vi "FMA1600A Meter Present.vi"(7 "Unit ID":string, 8 "error in (no error)":errorcluster, 9 "Meter Present":bool, 10 "Data Frame Format In":T2, 11 "VISA Refnum in":refnum<visa-resource-name>) -> (0 "error out":errorcluster, 2 "FMA1600A Gas Data":T3, 3 "Data Cluster":T1)   [LabVIEW 2023]
uses:
  Type Definitions/FMA1600A Data.ctl
  Alicat Gas Meter Driver/Sub-VIs/Data Frame.ctl
  Alicat Gas Meter Driver/Sub-VIs/Data Cluster.ctl
  Type Definitions/FMA1600A Commands.ctl
panel:
  # "Totalizer Timer"
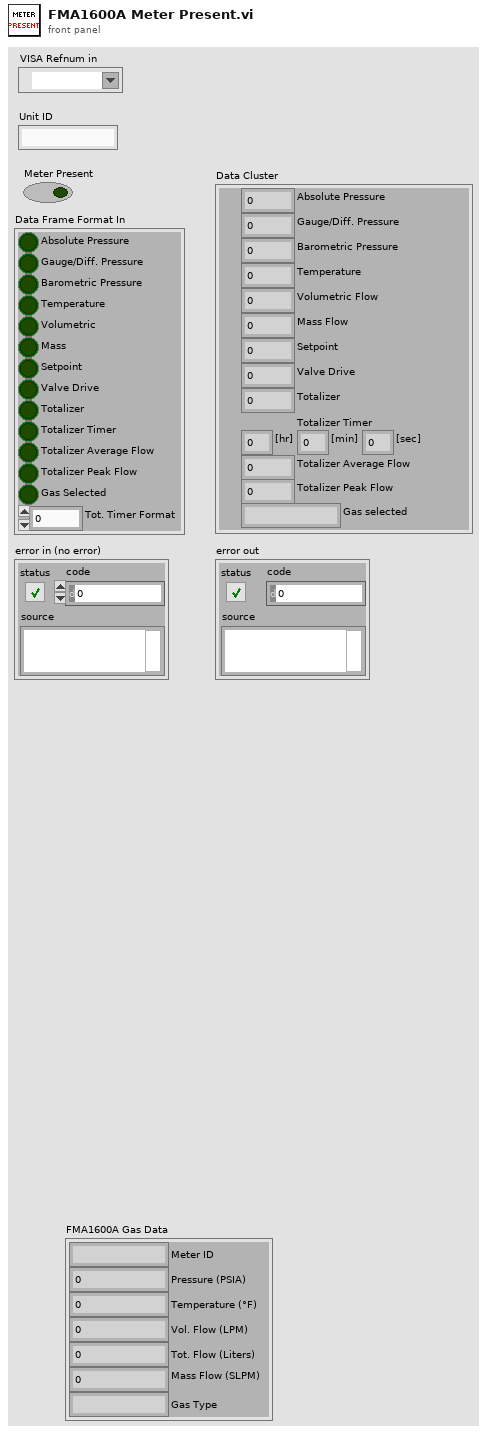
[diagram p1: front panel]
types:
  T1 = typedef "Data Cluster.ctl" = cluster{"Absolute Pressure":dbl, "Gauge/Diff. Pressure":dbl, "Barometric Pressure":dbl, "Temperature":dbl, "Volumetric Flow":dbl, "Mass Flow":dbl, "Setpoint":dbl, "Valve Drive":dbl, "Totalizer":dbl, "[hr]":dbl, "[min]":dbl, "[sec]":dbl, "Totalizer Average Flow":dbl, "Totalizer Peak Flow":dbl, "Gas selected":string}
  T2 = typedef "Data Frame.ctl" = cluster{"Absolute Pressure":bool, "Gauge/Diff. Pressure":bool, "Barometric Pressure":bool, "Temperature":bool, "Volumetric":bool, "Mass":bool, "Setpoint":bool, "Valve Drive":bool, "Totalizer":bool, "Totalizer Timer":bool, "Totalizer Average Flow":bool, "Totalizer Peak Flow":bool, "Gas Selected":bool, "Tot. Timer Format":u16}
  T3 = typedef "FMA1600A Data.ctl" = cluster{"Pressure (PSIA)":dbl, "Temperature (°F)":dbl, "Vol. Flow (LPM)":dbl, "Mass Flow (SLPM)":dbl, "Gas Type":string, "Tot. Flow (Liters)":dbl, "Meter ID":string}
  T4 = typedef "FMA1600A Commands.ctl" = string
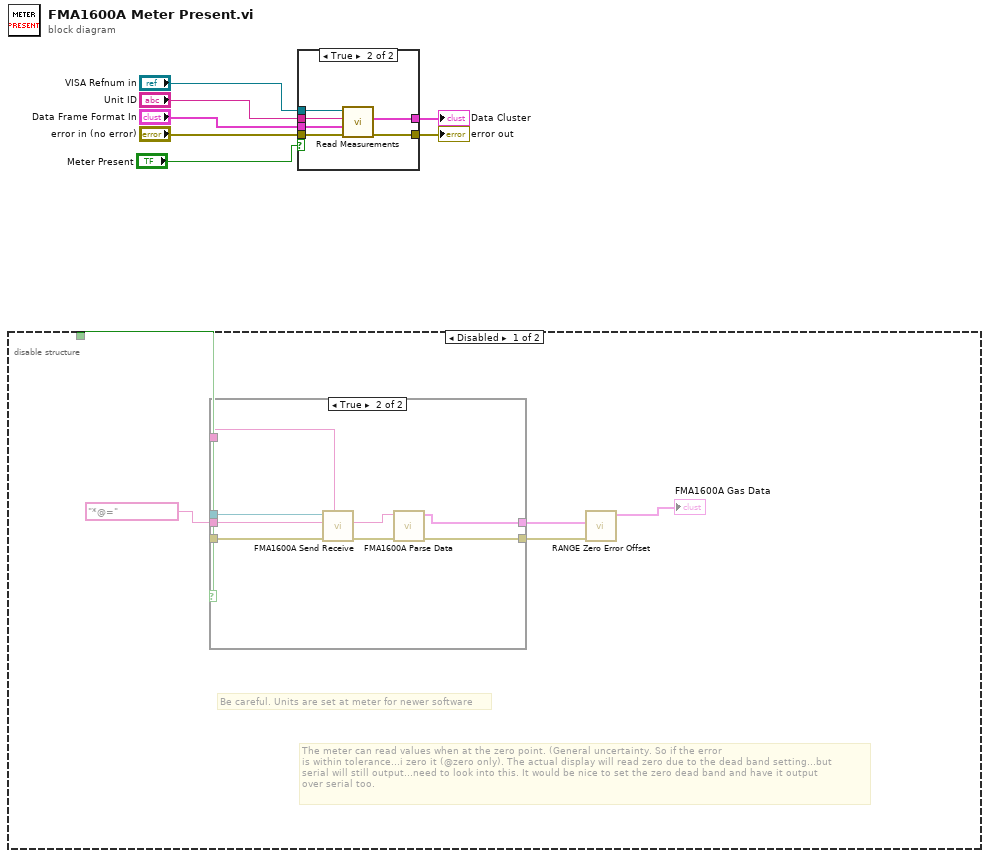
[diagram p0: block diagram]
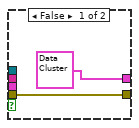
[diagram p2: hidden frame]
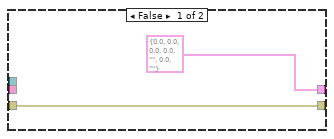
[diagram p3: hidden frame]
diagram:
  n1 = disable-structure shown="Disabled" {
    disable-tunnel: _ -> [w8 _]
    frame Disabled {
      # "Be careful. Units are set at meter for newer software"
      # "The meter can read values when at the zero point. (General uncertainty. So if the error\nis within tolerance...i zero it (@zero only). The actual display will read zero due to the dead band setting...but\nserial will still output...need to look into this. It would be nice to set the zero dead band and have it output\nover serial too."
      n2 = case shown="True" w8 {
        tunnel: [T3 {"Pressure (PSIA)"=0.0, "Temperature (°F)"=0.0, "Vol. Flow (LPM)"=0.0, "Mass Flow (SLPM)"=0.0, "Gas Type"="", "Tot. Flow (Liters)"=0.0, "Meter ID"=""} ("FMA1600A Gas Data") w27] -> w13
        tunnel: T4 "*@=" ("FMA1600A Commands") -> [_ w26]
        tunnel: [w19 w25] -> w15
        tunnel: [w19 w20] -> w10
        tunnel: [_ w24] -> w16
        tunnel: [_ w21] -> w17
        frame False {
        }
        frame True {
          n3 = call "FMA1600A Send Receive.vi"("Unit ID"=w21, "error in (no error)"=w25, "FMA1600A Commands"=w26, "VISA Refnum in"=w24) -> ("error out"=w23:errorcluster, "Raw FMA1600A Data"=w22:string)  [unwired: 5 in, 1 out]
          n4 = call "FMA1600A Parse Data.vi"("Error In"=w23, "Raw FMA1600A Data"=w22) -> ("Error Out"=w20:errorcluster, "FMA1600A Gas Data"=w27:T3)  [unwired: 7 in]
        }
      }
      n5 = call "RANGE Zero Error Offset.vi"("Error In"=w10, "FMA1600A Gas Data in"=w13) -> ("Error Out"=w9:errorcluster, "FMA1600A Gas Data out"=→"FMA1600A Gas Data":T3, "SLPM Error @ Zero"=w11:dbl)  [unwired: 7 in]
    }
    frame Enabled {
    }
  }
  n6 = case shown="True" "Meter Present" {
    tunnel: "Unit ID" -> [_ w35]
    tunnel: "VISA Refnum in" -> [_ w34]
    tunnel: "Data Frame Format In" -> [_ w33]
    tunnel: "error in (no error)" -> [w29 w32]
    tunnel: [w29 w31] -> w3
    tunnel: [T1 {"Absolute Pressure"=0.0, "Gauge/Diff. Pressure"=0.0, "Barometric Pressure"=0.0, "Temperature"=0.0, "Volumetric Flow"=0.0, "Mass Flow"=0.0, "Setpoint"=0.0, "Valve Drive"=0.0, "Totalizer"=0.0, "[hr]"=0.0, "[min]"=0.0, "[sec]"=0.0, "Totalizer Average Flow"=0.0, "Totalizer Peak Flow"=0.0, "Gas selected"=""} ("Data Cluster") w30] -> w2
    frame False {
    }
    frame True {
      n7 = call "Read Measurements.vi"("error in"=w32, "Data Frame Format In"=w33, "Unit ID (A)"=w35, "VISA Session In"=w34) -> ("error out"=w31:errorcluster, "Data Cluster"=w30:T1)  [unwired: 6 out]
    }
  }
  "error out" <- w3
  "Data Cluster" <- w2
